vi "test2-testModuleTurnsInvalidAPI.vi"(8 "error in (no error)":errorcluster, 11 "TestCase in":refnum<class "testcase-CSMNonCSMCallerSupportAPI.lvclass">) -> (0 "error out":errorcluster, 3 "TestCase out":refnum<class "testcase-CSMNonCSMCallerSupportAPI.lvclass">)   [LabVIEW 2017, in "testcase-CSMNonCSMCallerSupportAPI.lvclass"]
uses:
  testcase-CSMNonCSMCallerSupportAPI.lvclass
  InternalCluster.ctl
  GlobalVariable_CSMModeData.vi
  src/user.lib/_NEVSTOP/Communicable State Machine(CSM)/AdvanceAPI/CSM - List Modules.vi
  <vilib>/addons/_JKI Toolkits/VI Tester/TestCase.llb/TestCase.lvclass
  src/user.lib/_NEVSTOP/Communicable State Machine(CSM)/Communicable State Machine.lvlib
  C:/Program Files (x86)/National Instruments/LabVIEW 2017/vi.lib/addons/_JKI Toolkits/VI Tester/TestCase.llb/TestCase.lvclass
panel:
  in  "Stop":bool
  out "LoopCount":i32
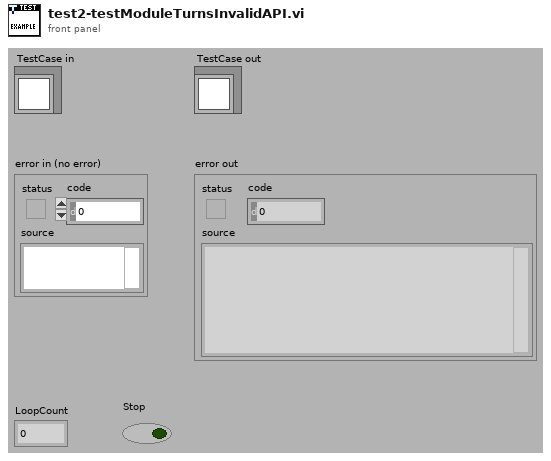
[diagram p1: front panel]
types:
  T1 = typedef "testcase-CSMNonCSMCallerSupportAPI.lvclass/InternalCluster.ctl" = cluster{"Mode":enum16{"Invalid", "Others", "WorkerAgent or Chain"}, "#Nodes":u32}
  T2 = enum16{"Invalid", "Others", "WorkerAgent or Chain"}
  T3 = typedef "Communicable State Machine.lvlib/_CSM_MODE.ctl" = enum16{"Not Exist", "Stand Alone", "CSM", "Worker", "Worker Agent", "Chain Node", "Chain"}
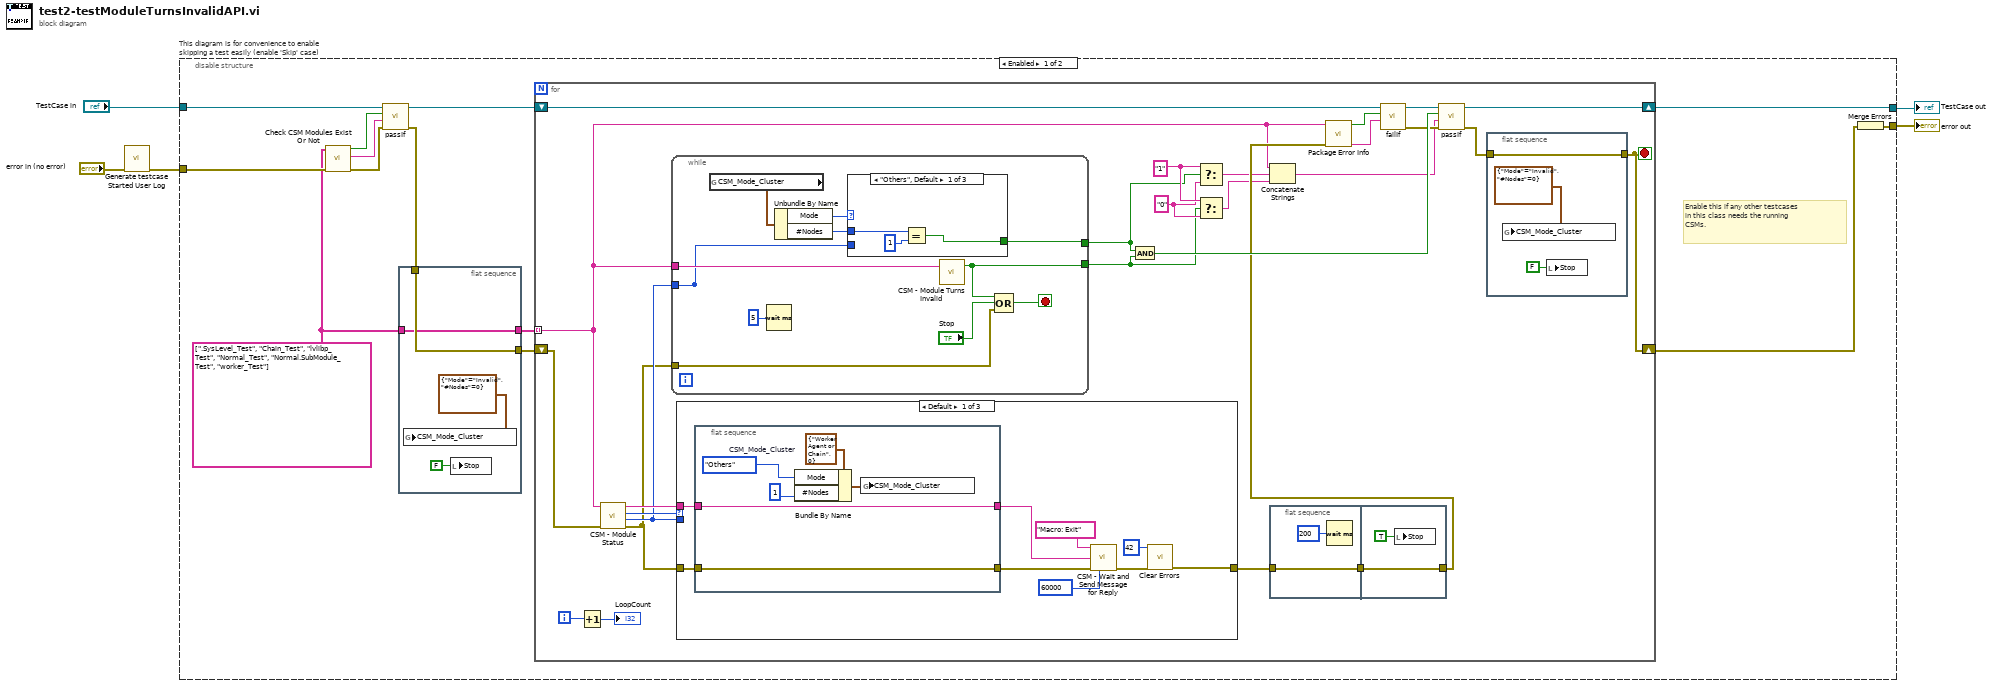
[diagram p0: block diagram]
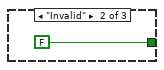
[diagram p2: hidden frame]
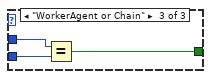
[diagram p3: hidden frame]
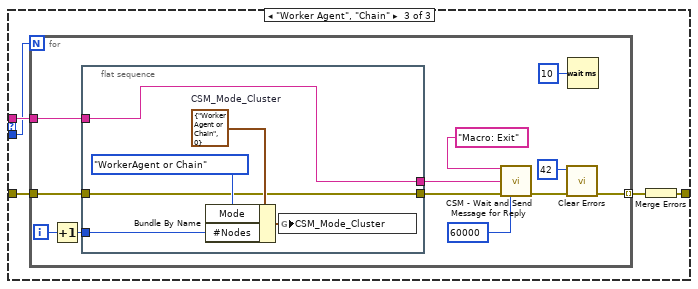
[diagram p5: hidden frame]
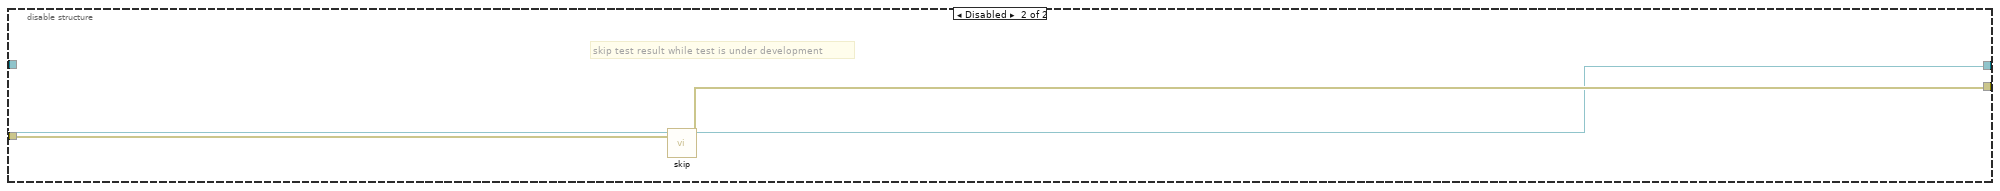
[diagram p6: hidden frame]
diagram:
  n1 = call "Generate testcase Started User Log.vi"("Error In"="error in (no error)") -> ("error out"=w1:errorcluster)  [unwired: 10 in]
  n2 = disable-structure "This diagram is for convenience to enable skipping a test easily (enable 'Skip' case)" shown="Enabled" {
    disable-tunnel: "TestCase in" -> [w14 w117]
    disable-tunnel: [w9 w115] -> w2
    disable-tunnel: [w7 w116] -> w4
    disable-tunnel: w1 -> [w12 w114]
    frame Enabled {
      w6 = string[] [".SysLevel_Test", "Chain_Test", "lvlibp_Test", "Normal_Test", "Normal.SubModule_Test", "worker_Test"] ("Module Names in All Scope")
      # "Enable this if any other testcases \nin this class needs the running\nCSMs."
      n3 = call "Check CSM Modules Exist Or Not.vi"("error in"=w12, "CSM names in"=w6) -> ("error out"=w16:errorcluster, "Debug string"=w17:string, "All Modules Exist?"=w18:bool)  [unwired: 7 in]
      n4 = call-dynamic "passIf.vi"("error in (no error)"=w16, "message (\"\")"=w17, "pass"=w18, "TestCase in"=w14) -> ("error out"=w15:errorcluster, "TestCase out"=w13:refnum<class "testcase-CSMNonCSMCallerSupportAPI.lvclass">)  [unwired: 6 in]
      n5 = flat-sequence {
        tunnel: [w20] -> w11
        tunnel: [w19] -> w10
        tunnel: w15 -> [w20]
        tunnel: w6 -> [w19]
        frame #0 {
          n6 = global write "GlobalVariable_CSMModeData.vi" "CSM_Mode_Cluster"(T1 {"Mode"=enum."Invalid", "#Nodes"=0} ("CSM_Mode_Cluster")) -> ()
          n7 = local write "Stop"(FALSE ("Stop")) -> ()
        }
      }
      n8 = for {
        shift-right: [w37] -> w8
        shift-left: w11 -> [w47]
        shift-right: [w44] -> w9
        shift-left: w13 -> [w34]
        tunnel: w10 -> [w24] mode=indexing
        i -> [w49]
        stop <- w37 stop-if-true
        w29 = "0"
        w30 = "1"
        n9 = Increment(x=w49) -> (x+1=→"LoopCount":i32)
        n10 = call "CSM - Module Status.vi"("Error In"=w47, "CSM Name"=w24) -> ("error out"=w38:errorcluster, "#Nodes"=w40:i32, "Mode"=w46:T3, "CSM Name (Dup)"=w45:string)  [unwired: 5 in, 1 out]
        n11 = while {
          tunnel: w24 -> [w64]
          tunnel: [w58] -> _
          tunnel: w40 -> [w58]
          tunnel: [w57] -> w25
          tunnel: [w56] -> w26
          tunnel: w38 -> [w55]
          stop <- w62 stop-if-true
          n12 = global read "GlobalVariable_CSMModeData.vi" "CSM_Mode_Cluster"() -> (w61:T1)
          n13 = Wait (ms)(milliseconds to wait=u32 5) -> ()  [unwired: 1 out]
          n14 = Unbundle By Name(w61) -> ("Mode"=w60:T2, "#Nodes"=w59:u32)
          n15 = case shown="\"Others\", Default" w60 {
            tunnel: [w67 FALSE w70] -> w56
            tunnel: w59 -> [w66 _ w71]
            tunnel: w58 -> [_ _ w69]
            frame "Others", Default {
              n16 = Equal?(x=w66, y=1) -> (x = y?=w67:bool)
            }
            frame "Invalid" {
            }
            frame "WorkerAgent or Chain" {
              n17 = Equal?(x=w71, y=w69) -> (x = y?=w70:bool)
            }
          }
          n18 = call "CSM - Module Turns Invalid.vi"("CSM Name"=w64) -> ("Turn Invalid (Exit)?"=w57:bool)  [unwired: 2 in]
          n19 = Compound Arithmetic op=OR(w57, "Stop", w55) -> (w62:bool)
        }
        n20 = case shown="Default" w46 {
          tunnel: w38 -> [w77 w90 w95]
          tunnel: w40 -> [_ _ w93]
          tunnel: w45 -> [w79 _ w94]
          tunnel: [w81 w90 w92] -> w42
          frame Default {
            n21 = flat-sequence {
              tunnel: w79 -> [w85]
              tunnel: [w85] -> w78
              tunnel: w77 -> [w84]
              tunnel: [w84] -> w76
              frame #0 {
                w89 = T1 {"Mode"=enum."WorkerAgent or Chain", "#Nodes"=0}  # CSM_Mode_Cluster
                n22 = Bundle By Name(cluster=w89, "Mode"=T2."Others", "#Nodes"=u32 1) -> (w88:T1)
                n23 = global write "GlobalVariable_CSMModeData.vi" "CSM_Mode_Cluster"(w88) -> ()
              }
            }
            n24 = call "CSM - Wait and Send Message for Reply.vi"("State"="Macro: Exit", "Target Module"=w78, "Error In (No Error)"=w76, "Response Timeout (-2 Using Global Settings)"=60000) -> ("error out"=w82:errorcluster)  [unwired: 8 in, 3 out]
            n25 = call <vilib>:"Clear Errors.vi"("error in (no error)"=w82, "specific error code to clear (0: all)"=42) -> ("error out"=w81:errorcluster)  [unwired: 4 in, 1 out]
          }
          frame "Not Exist" {
          }
          frame "Worker Agent", "Chain" {
            n26 = for {
              N: w93 -> [_]
              tunnel: w94 -> [w98]
              tunnel: w95 -> [w100]
              tunnel: [w103] -> w91 mode=indexing
              i -> [w106]
              n27 = Increment(x=w106) -> (x+1=w105:i32)
              n28 = flat-sequence {
                tunnel: w105 -> [w111]
                tunnel: w100 -> [w109]
                tunnel: [w109] -> w99
                tunnel: w98 -> [w108]
                tunnel: [w108] -> w97
                frame #0 {
                  w113 = T1 {"Mode"=enum."WorkerAgent or Chain", "#Nodes"=0}  # CSM_Mode_Cluster
                  n29 = Bundle By Name(cluster=w113, "Mode"=T2."WorkerAgent or Chain", "#Nodes"=w111) -> (w112:T1)
                  n30 = global write "GlobalVariable_CSMModeData.vi" "CSM_Mode_Cluster"(w112) -> ()
                }
              }
              n31 = call "CSM - Wait and Send Message for Reply.vi"("State"="Macro: Exit", "Target Module"=w97, "Error In (No Error)"=w99, "Response Timeout (-2 Using Global Settings)"=60000) -> ("error out"=w104:errorcluster)  [unwired: 8 in, 3 out]
              n32 = call <vilib>:"Clear Errors.vi"("error in (no error)"=w104, "specific error code to clear (0: all)"=42) -> ("error out"=w103:errorcluster)  [unwired: 4 in, 1 out]
              n33 = Wait (ms)(milliseconds to wait=u32 10) -> ()  [unwired: 1 out]
            }
            n34 = Merge Errors(w91) -> (w92:errorcluster)
          }
        }
        n35 = And(x=w26, y=w25) -> (x .and. y?=w39:bool)
        n36 = Select(t=w30, s=w26, f=w29) -> (s? t:f=w28:string)
        n37 = Select(t=w30, s=w25, f=w29) -> (s? t:f=w27:string)
        n38 = flat-sequence {
          tunnel: w42 -> [w51]
          tunnel: [w51] -> w41
          tunnel: [w53] -> w31
          tunnel: w41 -> [w53]
          frame #0 {
            n39 = Wait (ms)(milliseconds to wait=u32 200) -> ()  [unwired: 1 out]
          }
          frame #1 {
            n40 = local write "Stop"(TRUE ("Stop")) -> ()
          }
        }
        n41 = Concatenate Strings(w24, w28, w27) -> (w23:string)
        n42 = call "Package Error Info.vi"("error in"=w31, "String in"=w24) -> ("packed error info out"=w35:string, "error status"=w36:bool)  [unwired: 8 in]
        n43 = call-dynamic "failIf.vi"("message (\"\")"=w35, "fail"=w36, "TestCase in"=w34) -> ("error out"=w32:errorcluster, "TestCase out"=w33:refnum<class "testcase-CSMNonCSMCallerSupportAPI.lvclass">)  [unwired: 7 in]
        n44 = call-dynamic "passIf.vi"("error in (no error)"=w32, "message (\"\")"=w23, "pass"=w39, "TestCase in"=w33) -> ("error out"=w43:errorcluster, "TestCase out"=w44:refnum<class "testcase-CSMNonCSMCallerSupportAPI.lvclass">)  [unwired: 6 in]
        n45 = flat-sequence {
          tunnel: w43 -> [w73]
          tunnel: [w73] -> w37
          frame #0 {
            n46 = global write "GlobalVariable_CSMModeData.vi" "CSM_Mode_Cluster"(T1 {"Mode"=enum."Invalid", "#Nodes"=0} ("CSM_Mode_Cluster")) -> ()
            n47 = local write "Stop"(FALSE ("Stop")) -> ()
          }
        }
      }
      n48 = Merge Errors(w8) -> (w7:errorcluster)
    }
    frame Disabled {
      # "skip test result while test is under development"
      n49 = call <vilib>:"skip.vi"("error in (no error)"=w114, "TestCase in"=w117) -> ("error out"=w116:errorcluster, "TestCase out"=w115:refnum<class "testcase-CSMNonCSMCallerSupportAPI.lvclass">)  [unwired: 8 in]
    }
  }
  "error out" <- w4
  "TestCase out" <- w2
